vi "ADVM - AC Characteristics 2 Channel Measurements.vi"() -> ()   [LabVIEW 2021]
uses:
  <vilib>/PDM Acquisition Toolkit/shared/controls/i2s frame size.ctl
  <vilib>/PDM Acquisition Toolkit/shared/controls/PCM Data Format Configuration.ctl
  <vilib>/PDM Acquisition Toolkit/shared/controls/Digital Edge.ctl
  <vilib>/PDM Acquisition Toolkit/shared/controls/PCM Bit Endianness.ctl
  <vilib>/PDM Acquisition Toolkit/shared/controls/PCM Data Justification.ctl
  <vilib>/PDM Acquisition Toolkit/shared/controls/PCM Frame Sync Control.ctl
  <vilib>/PDM Acquisition Toolkit/host/Classes/Tasks/PDM Tasks/Controls/Acquisition Mode.ctl
  <vilib>/addons/_NISVFA/_Shared subVIs/Controls/svc_Window.ctl
  <vilib>/addons/_NISVFA/_Shared subVIs/Common/SVL Set dB Reference (N Ch - 1 Ref).vi
  <vilib>/addons/Sound and Vibration/svt_Level/SVL AC & DC Level (Time) (N Ch).vi
  <vilib>/addons/Sound and Vibration/svt_Single Tone Measurements/SVT Spurious Free Dynamic Range (Frequency) (1 Ch).vi
  <vilib>/addons/_NISVFA/_Spectrum Processing/SVFA Unit Conversion (Complex) (1 Ch).vi
  <vilib>/addons/_NISVFA/_Spectrum Processing/SVFA Get Spectrum Subset (1 Ch).vi
  <vilib>/addons/_NISVFA/_Shared subVIs/Common/SVL Set dB Reference (1 Ch).vi
  <vilib>/addons/Sound and Vibration/svt_Level/SVL AC & DC Level (Time) (1 Ch).vi
  <vilib>/addons/_NISVFA/_Spectrum Processing/SVFA Get Spectrum Subset (Complex) (1 Ch).vi
  <vilib>/addons/_NISVFA/_Shared subVIs/Common/svc_Window Parameters.vi
  <vilib>/addons/_NISVFA/_Shared subVIs/Common/svc_Extract Single Tone Information (complex).vi
  <vilib>/addons/_NISVFA/_Shared subVIs/Common/svc_Check Frequency Range in Spectrum.vi
  <vilib>/addons/_NISVFA/_Spectrum Processing/SVFA Spectrum Peak Search.vi
  <vilib>/addons/_NISVFA/_Spectrum Processing/SVFA Spectrum Peak Search (1 Ch).vi
  <vilib>/addons/_NISVFA/_Shared subVIs/Common/svc_Spectrum Units.vi
  <vilib>/addons/_NISVFA/_Shared subVIs/Common/svc_Log View for Spectrum (1Ch).vi
  <vilib>/addons/_NISVFA/_Spectrum Processing/SVFA Unit Conversion (1 Ch).vi
  <vilib>/addons/_NISVFA/_Shared subVIs/Common/svc_Complex Datatype Defaults.vi
  <vilib>/addons/_NISVFA/_Shared subVIs/Common/svc_Build Unit Label for Frequency Range.vi
  <vilib>/addons/_NISVFA/_Shared subVIs/Common/SVL Set dB Reference (variant).vi
  <vilib>/addons/_NISVFA/_Shared subVIs/Common/svc_Get SV Channel Info.vi
  <vilib>/Analysis/baseanly.llb/Mean.vi
  <vilib>/Analysis/baseanly.llb/Mean (DBL).vi
  <vilib>/addons/_NISVFA/_Shared subVIs/Windowing/svfa_Scaled Time Domain Window (Array).vi
  <vilib>/addons/_NISVFA/_Spectrum Processing/SVFA Get Tone Amplitude and Phase (1 Ch).vi
  <vilib>/addons/_NISVFA/_Spectrum Processing/subVIs/svfa_Compute Complex Spectrum for Export.vi
  <vilib>/addons/_NISVFA/_Shared subVIs/Common/svc_Check Frequency Range in Bandwidth.vi
  <vilib>/addons/_NISVFA/_Shared subVIs/Common/svc_Convert Start and Stop to Start Index and Length.vi
  <vilib>/addons/_NISVFA/_Spectrum Processing/subVIs/svfa_Spectrum Peak Search.vi
  <vilib>/addons/_NISVFA/_Shared subVIs/Common/svc_Format Value (DBL).vi
  <vilib>/addons/_NISVFA/_Shared subVIs/Common/svc_Get Weighting Enum and Labels.vi
  <vilib>/addons/_NISVFA/_Shared subVIs/Common/svc_Engineering Units to Unit Label.vi
  <vilib>/addons/_NISVFA/_Shared subVIs/Common/svc_Surround NonAlpha String with Parentheses.vi
  <vilib>/dlg_ctls.llb/Space Constant.vi
  <vilib>/addons/_NISVFA/_Shared subVIs/Common/svc_Unwrap Phase.vi
  <vilib>/addons/_NISVFA/_Shared subVIs/Common/svc_Convert Spectrum Array to dB.vi
  <vilib>/addons/_NISVFA/_Spectrum Processing/subVIs/svfa_Conversion Utility (spectrum info).vi
  <vilib>/addons/_NISVFA/_Shared subVIs/Common/svc_Unit Label to Engineering Units.vi
  <vilib>/addons/_NISVFA/_Spectrum Processing/subVIs/svfa_Spectrum Info Window to windowTd Type Def.vi
  <vilib>/Analysis/4window.llb/Force Window.vi
  <vilib>/Analysis/4window.llb/Force Window (DBL).vi
  <vilib>/Analysis/4window.llb/Exponential Window.vi
  <vilib>/Analysis/4window.llb/Exponential Window (DBL).vi
  <vilib>/addons/_NISVFA/_Spectrum Processing/subVIs/svfa_Window Frequency Response.vi
  <vilib>/addons/_NISVFA/_Spectrum Processing/subVIs/svfa_Window Frequency Response (double array).vi
  <vilib>/Analysis/baseanly.llb/Dot Product.vi
  <vilib>/Analysis/baseanly.llb/Complex Dot Product.vi
  <vilib>/addons/_NISVFA/_Spectrum Processing/subVIs/svfa_Peak Rough Search Indices.vi
  <vilib>/addons/_NISVFA/_Shared subVIs/Common/svc_Unit Label Lexical Class.vi
  <vilib>/addons/_NISVFA/_Spectrum Processing/subVIs/svfa_Peak to RMS to Peak2Peak.vi
  <vilib>/addons/_NISVFA/_Spectrum Processing/subVIs/svfa_Mag to Mag2.vi
  <vilib>/addons/_NISVFA/_Spectrum Processing/subVIs/svfa_Linear to dB.vi
  <vilib>/addons/_NISVFA/_Spectrum Processing/subVIs/svfa_dBrefA to dBrefB.vi
  <vilib>/addons/_NISVFA/_Spectrum Processing/subVIs/svfa_Spectrum to Spectral Density.vi
  <vilib>/addons/_NISVFA/_Spectrum Processing/subVIs/svfa_Rect Window Frequency Response.vi
  <vilib>/addons/_NISVFA/_Spectrum Processing/subVIs/svfa_Cosine Window Coefficients.vi
  <vilib>/PDM Acquisition Toolkit/host/API/Public/Create Tasks/Create PCM Input Task.vi
  <vilib>/PDM Acquisition Toolkit/host/API/Public/Configure/Timing/Configure Timing - PCM Input Slave.vi
  <vilib>/PDM Acquisition Toolkit/host/API/Public/Configure/PDM Channel/Configure Microphone Sensitivity FSPA - PCM Input Task.vi
  <vilib>/DAQmx/create/channels.llb/DAQmx Create Channel (AO-FuncGen).vi
  <vilib>/PDM Acquisition Toolkit/host/API/Public/Commit/Commit PCM Input Task.vi
  <vilib>/PDM Acquisition Toolkit/host/API/Public/Start/Start PCM Input Task.vi
  <vilib>/PDM Acquisition Toolkit/host/API/Public/Read/Read PCM Input Waveform.vi
  <vilib>/PDM Acquisition Toolkit/host/API/Public/Clear/Clear PCM Input Task.vi
  <vilib>/addons/Sound and Vibration/svt_Weighting/SVT Weighting Filter (N Ch).vi
  <vilib>/addons/_NISVFA/_Shared subVIs/Common/svc_Caller VI Returned in Error Source.vi
  <vilib>/addons/_NISVFA/_Shared subVIs/Common/svc_Get Window Info.vi
  <vilib>/Analysis/0measdsp.llb/Scaled Time Domain Window.vi
  <vilib>/Analysis/0measdsp.llb/Scaled Time Domain Window (DBL).vi
  <vilib>/Utility/error.llb/Error Cluster From Error Code.vi
  <vilib>/Analysis/baseanly.llb/Std Deviation and Variance.vi
  <vilib>/addons/Sound and Vibration/svt_Single Tone Measurements/SVT Gain (Time) (1 Ch).vi
  <vilib>/addons/Sound and Vibration/svt_Distortion/SVT SNR without Harmonics (Frequency) (1 Ch).vi
  <vilib>/addons/Sound and Vibration/svt_Single Tone Measurements/SVT Dynamic Range (Frequency) (1 Ch).vi
  <vilib>/addons/Sound and Vibration/svt_Distortion/subVIs/sv_Check Data Valid (Audio) (1 Ch).vi
  <vilib>/addons/_NISVFA/_Shared subVIs/Common/svc_Convert Frequency to Frequency String.vi
  <vilib>/Analysis/4window.llb/window parameters.vi
  <vilib>/Analysis/4window.llb/Window Properties.vi
  <vilib>/Analysis/4window.llb/Window Properties by Name.vi
  <vilib>/addons/_NISVFA/_Spectrum Processing/subVIs/svfa_Spectrum Peak Tone Search and Estimation (complex).vi
  <vilib>/measure/masignal.llb/Tones and Noise Waveform.vi
  <vilib>/addons/_NISVFA/_Shared subVIs/Common/svc_FFT with Window.vi
  <vilib>/Analysis/1siggen.llb/Square Wave.vi
  <vilib>/addons/_NISVFA/_Spectrum Processing/subVIs/svfa_Three Finger Peak Search.vi
  <vilib>/addons/Sound and Vibration/svt_Distortion/subVIs/sv_Peak View Amplitude (1 Ch).vi
  <vilib>/PDM Acquisition Toolkit/host/Classes/Tasks/PDM Tasks/PDM Task.lvclass
  <vilib>/PDM Acquisition Toolkit/host/API/PDM Acquisition Toolkit.lvlib
  <vilib>/addons/Sound and Vibration/svt_Single Tone Measurements/SoundVib_SingleTone.lvlib
  <vilib>/addons/Sound and Vibration/svt_Distortion/SoundVib_Distortion.lvlib
  <vilib>/PDM Acquisition Toolkit/shared/PDM Shared.lvlib
  <vilib>/addons/Sound and Vibration/svt_Weighting/SoundVib_ABCWeighting.lvlib
  <vilib>/PDM Acquisition Toolkit/host/API/Public/Configure/Timing/Configure Timing - I2S Input Slave.vi
  <vilib>/PDM Acquisition Toolkit/host/API/Public/Create Tasks/Create I2S Input Task.vi
  <vilib>/PDM Acquisition Toolkit/host/Classes/Tasks/I2S Input/I2S Input Task.lvclass
  <vilib>/PDM Acquisition Toolkit/host/Classes/Tasks/PCM Input/PCM Input Task.lvclass
panel:
  in  "DSG resource name":string="4468/ao0:1"
  in  "WEIGHTING":T1(ring)
  in  "DUT FULL SCALE":dbl=3.16 format="%.3p"
  out "error out":errorcluster
  out "Sampling Rate":dbl=192000.0 format="%#_6p"
  out "MeasTable":string[][](table)
  in  "I2S Number of Words":u32=19200 caption="NO OF WORDS"
  in  "I2S Word Length":u32=24 caption="WORD LENGTH"
  in  "I2S Clock Rate":u32=12288000 caption="CLOCK RATE"
  in  "THD Maximum Harmonic":u32=9 caption="MAX HARMONIC"
  in  "Measurement Band Stop":dbl=20000.0 caption="BAND STOP" format="%#_6pHz"
  in  "Measurement Band Start":dbl=20.0 caption="BAND START" format="%#_6pHz"
  in  "DSG amplitude":dbl=1.0 caption="AMPLITUDE" format="%#_6pV"
  in  "DSG frequency":dbl=1000.0 caption="FREQUENCY" format="%#_6pHz"
  in  "Mic sensitivity (FS/Pa)":dbl=0.34762 caption="SENSITIVITY" format="%.3fFS/Pa"
  in  "I2S Channel List":string="7820\\PCMi 0" caption="CHANNEL LIST"
  out "MeasGraphs":enum32{"Frequency Domain", "Time Domain"}(tab)
  out "FrequencyDomain":cluster{"x0":dbl, "dx":dbl, "magnitude":dbl[]}[](graph) caption="AC"
  out "TimeDomain":waveform(dbl)[](graph) caption="AC"
  # "Measurement"
  # "Analog Source"
  # "Protocol Setting"
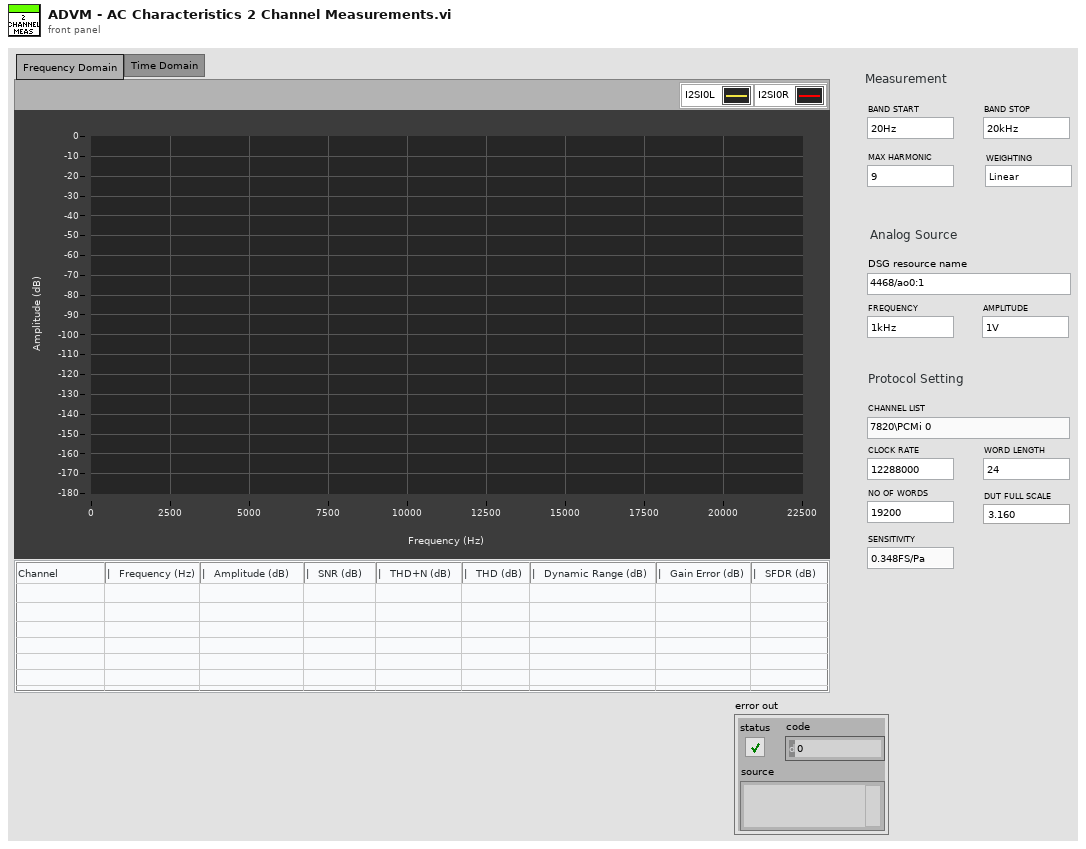
[diagram p1: front panel]
types:
  T1 = enum16{"Linear", "A-weighting", "B-weighting", "C-weighting"}
  T2 = cluster{"band start (Hz)":dbl, "band stop (Hz)":dbl}
  T3 = typedef "PDM Shared.lvlib/i2s frame size.ctl" = enum16{"32bits", "64bits"}
  T4 = cluster{"frequency range":cluster{"band start (Hz)":dbl, "band stop (Hz)":dbl}, "THD maximum harmonic":i32, "amplitude":dbl, "frequency (Hz)":dbl, "microphone sensitivity (FS/Pa)":dbl, "number of words":i32, "channel list":string, "logic level":enum16{"3.3 V", "1.8 V", "1.2 V"}, "I2S serial clock rate 2":u32, "frame size":T3, "word length":u32, "Data Latch at SCK cycle":u8, "Playback .WAV File?":bool, "Record .WAV File?":bool, "Record wave file path":path, "Playback .WAV file path":path, "number of channels":i32, "DUT full scale (V pk)":dbl, "output channel":tag[]}
  T5 = typedef "PDM Shared.lvlib/PCM Frame Sync Control.ctl" = cluster{"Frame Length":u16, "Frame Sync Pulse Width":u16, "Bit Clock Edge  Sync":T6}
  T6 = typedef "PDM Shared.lvlib/Digital Edge.ctl" = enum8{"Rising", "Falling"}
  T7 = typedef "PDM Shared.lvlib/PCM Data Format Configuration.ctl" = cluster{"Frame Sync Edge for Channel 0":T6, "Channel Count Per Frame":u8, "Channel Length":u16, "Bit Depth":u8, "Channel 0 Offset":u16, "Endianness":T8, "Data Justification":T9}
  T8 = typedef "PDM Shared.lvlib/PCM Bit Endianness.ctl" = enum16{"MSB First", "LSB First"}
  T9 = typedef "PDM Shared.lvlib/PCM Data Justification.ctl" = enum16{"Left Justified", "Right Justified"}
  T10 = typedef "PDM Acquisition Class Library.lvlib/PDM Task.lvclass/Acquisition Mode.ctl" = enum16{"Finite", "Continuous"}
  T11 = cluster{"linear/dB":enum16{"no change", "linear", "dB"}, "dB reference (0: no change)":dbl, "power/magnitude":enum16{"no change", "power", "magnitude"}, "view":enum16{"no change", "rms", "peak", "peak-peak"}}
  T12 = enum16{"no change", "spectrum", "spectral density"}
  T13 = cluster{"gain units":enum16{"dB", "linear ratio"}, "detected fundamental amplitude units":enum16{"EU rms", "EU peak", "EU peak-peak"}}
  T14 = cluster{"SNR units":enum16{"dB", "linear ratio", "%"}, "detected fundamental amplitude units":enum16{"EU rms", "EU peak", "EU peak-peak"}}
  T15 = typedef "PDM Acquisition Class Library.lvlib/I2S Input Task.lvclass/DVR I2S Input Task.ctl" = refnum<data-value>
  T16 = typedef "PDM Acquisition Class Library.lvlib/PCM Input Task.lvclass/DVR PCM Input Task.ctl" = refnum<data-value>
  T17 = typedef "svc_Window.ctl" = u32
  T18 = typedef "svc_Spectrum Info.ctl" = cluster{"channel name":string, "description":string, "x-axis units":T19, "spectral info":cluster{"spectrum type":T20, "linear/dB":enum16{"linear", "dB"}, "window":u16, "window size":i32, "FFT size":i32}, "engineering units":T21, "custom label":string, "dB reference [EU]":dbl, "peak units":enum16{"rms", "peak", "peak-peak"}, "weighting filter":T22, "spectral density?":bool, "unit label":string, "spectrum skewed?":bool, "complimentary spectrum units":T23}
  T19 = typedef "svc_X-Axis Units.ctl" = u16
  T20 = typedef "svc_Spectrum Type.ctl" = enum16{"FFT Spectrum [complex]", "Amplitude [Magnitude]", "Power [Magnitude^2]", "Cross Spectrum [complex]", "Frequency Response [Complex]"}
  T21 = typedef "svc_Engineering Units Text Ring.ctl" = u16
  T22 = typedef "svc_Weighting Filter Text Ring.ctl" = u16
  T23 = typedef "svc_Complimentary Spectrum Units.ctl" = enum16{"none", "radians", "degrees", "cycles", "imaginary"}
  T24 = cluster{"complex spectrum response":cluster{"f0":dbl, "df":dbl, "complex spectrum":cdb[]}, "spectrum info":T18}
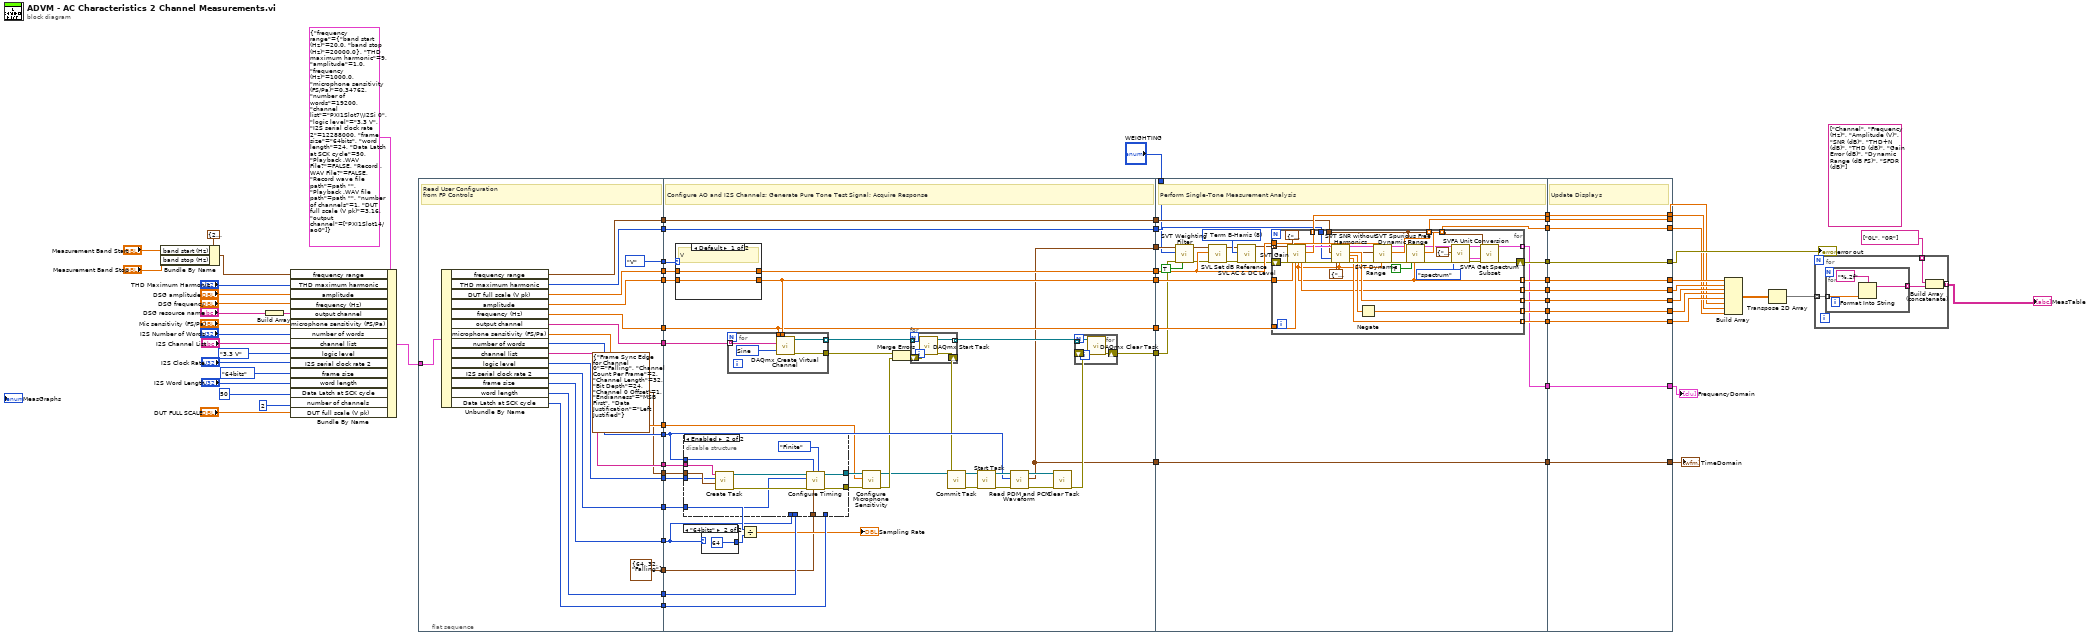
[diagram p0: block diagram]
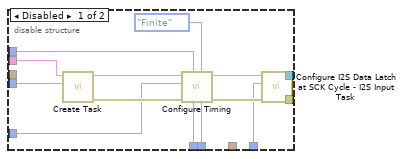
[diagram p2: hidden frame]
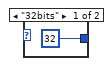
[diagram p3: hidden frame]
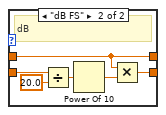
[diagram p4: hidden frame]
diagram:
  (unwired) string[] ["Channel", "Frequency (Hz)", "Amplitude (V)", "SNR (dB)", "THD+N (dB)", "THD (dB)", "Gain Error (dB)", "Dynamic Range (dB FS)", "SFDR (dB)"] ("MeasTable")
  n1 = Bundle By Name(cluster=T2 {"band start (Hz)"=20.0, "band stop (Hz)"=20000.0} ("frequency range"), "band start (Hz)"="Measurement Band Start", "band stop (Hz)"="Measurement Band Stop") -> (w39:T2)
  n2 = Build Array("DSG resource name") -> (w6:string[])
  n3 = Bundle By Name(cluster=T4 {"frequency range"={"band start (Hz)"=20.0, "band stop (Hz)"=20000.0}, "THD maximum harmonic"=9, "amplitude"=1.0, "frequency (Hz)"=1000.0, "microphone sensitivity (FS/Pa)"=0.34762, "number of words"=19200, "channel list"="PXI1Slot7\\I2Si 0", "logic level"=enum."3.3 V", "I2S serial clock rate 2"=12288000, "frame size"=enum."64bits", "word length"=24, "Data Latch at SCK cycle"=50, "Playback .WAV File?"=FALSE, "Record .WAV File?"=FALSE, "Record wave file path"=path "", "Playback .WAV file path"=path "", "number of channels"=1, "DUT full scale (V pk)"=3.16, "output channel"=["PXI1Slot14/ao0"]}, "frequency range"=w39, "THD maximum harmonic"="THD Maximum Harmonic", "amplitude"="DSG amplitude", "frequency (Hz)"="DSG frequency", "output channel"=w6, "microphone sensitivity (FS/Pa)"="Mic sensitivity (FS/Pa)", "number of words"="I2S Number of Words", "channel list"="I2S Channel List", "logic level"=enum16{"3.3 V", "1.8 V", "1.2 V"}."3.3 V" ("I2S Logic Level"), "I2S serial clock rate 2"="I2S Clock Rate", "frame size"=enum16{"32bits", "64bits"}."64bits" ("I2S Frame Size"), "word length"="I2S Word Length", "Data Latch at SCK cycle"=u8 50 ("I2S Data Latch at SCK Cycle"), "number of channels"=2, "DUT full scale (V pk)"="DUT FULL SCALE") -> (w26:T4)
  n4 = flat-sequence {
    tunnel: [w88] -> w73
    tunnel: [w85] -> w72
    tunnel: [w84] -> w71
    tunnel: [w87] -> w70
    tunnel: [w86] -> w69
    tunnel: [enum16{"V", "dB FS"}."V" ("amplitude units")] -> w68
    tunnel: [w79] -> w67
    tunnel: [w80] -> w66
    tunnel: [w76] -> w65
    tunnel: [w82] -> w64
    tunnel: [w77] -> w63
    tunnel: [w78] -> w62
    tunnel: [w81] -> w61
    tunnel: [w83] -> w45
    tunnel: w26 -> [w90]
    tunnel: [w89] -> w25
    tunnel: [T7 {"Frame Sync Edge for Channel 0"=enum."Falling", "Channel Count Per Frame"=2, "Channel Length"=32, "Bit Depth"=24, "Channel 0 Offset"=1, "Endianness"=enum."MSB First", "Data Justification"=enum."Left Justified"} ("PCM data configuration")] -> w2
    tunnel: [T5 {"Frame Length"=64, "Frame Sync Pulse Width"=32, "Bit Clock Edge  Sync"=enum."Falling"} ("Frame Sync Clock Control")] -> w1
    tunnel: w73 -> [w126]
    tunnel: w72 -> [w119]
    tunnel: w71 -> [w124]
    tunnel: w70 -> [w129]
    tunnel: w69 -> [w128]
    tunnel: w68 -> [w125]
    tunnel: [w130] -> w60
    tunnel: [w127] -> w59
    tunnel: [w126] -> w58
    tunnel: [w123] -> w57
    tunnel: [w119] -> w56
    tunnel: [w99] -> w55
    tunnel: [w117] -> w54
    tunnel: w67 -> [w109]
    tunnel: w66 -> [w108]
    tunnel: w65 -> [w107]
    tunnel: w64 -> [w106]
    tunnel: w63 -> [w105]
    tunnel: w62 -> [w104]
    tunnel: w61 -> [w103]
    tunnel: w45 -> [w96]
    tunnel: w25 -> [w130]
    tunnel: [w99] -> w21
    tunnel: w2 -> [w93]
    tunnel: w1 -> [w92]
    tunnel: [w200] -> w53
    tunnel: [w199] -> w52
    tunnel: [w190] -> w51
    tunnel: [w198] -> w50
    tunnel: [w197] -> w49
    tunnel: [w196] -> w48
    tunnel: [w195] -> w47
    tunnel: [w189] -> w46
    tunnel: w60 -> [w188]
    tunnel: w59 -> [w202]
    tunnel: w58 -> [w193]
    tunnel: w57 -> [w201]
    tunnel: w56 -> [w194]
    tunnel: w55 -> [w186]
    tunnel: w54 -> [w184]
    tunnel: [w191] -> w22
    tunnel: w21 -> [w191]
    tunnel: [w187] -> w20
    tunnel: "WEIGHTING" -> [w182]
    tunnel: [w179] -> w4
    tunnel: w53 -> [w243]
    tunnel: w52 -> [w242]
    tunnel: w51 -> [w250]
    tunnel: w50 -> [w244]
    tunnel: w49 -> [w245]
    tunnel: w48 -> [w246]
    tunnel: w47 -> [w247]
    tunnel: w46 -> [w248]
    tunnel: [w250] -> w44
    tunnel: [w249] -> w23
    tunnel: w22 -> [w249]
    tunnel: w20 -> [w241]
    tunnel: [w248] -> w19
    tunnel: [w247] -> w18
    tunnel: [w246] -> w17
    tunnel: [w245] -> w16
    tunnel: [w244] -> w15
    tunnel: [w243] -> w14
    tunnel: [w242] -> w13
    tunnel: [w241] -> w12
    tunnel: w4 -> [w240]
    tunnel: [w240] -> w3
    frame #0 {
      # "Read User Configuration\nfrom FP Controls"
      n5 = Unbundle By Name(w90) -> ("frequency range"=w89:T2, "THD maximum harmonic"=w88:i32, "DUT full scale (V pk)"=w87:dbl, "amplitude"=w86:dbl, "frequency (Hz)"=w85:dbl, "output channel"=w84:tag[], "microphone sensitivity (FS/Pa)"=w83:dbl, "number of words"=w82:i32, "channel list"=w81:string, "logic level"=w80:enum16{"3.3 V", "1.8 V", "1.2 V"}, "I2S serial clock rate 2"=w79:u32, "frame size"=w78:T3, "word length"=w77:u32, "Data Latch at SCK cycle"=w76:u8)
    }
    frame #1 {
      # "Configure AO and I2S Channels; Generate Pure Tone Test Signal; Acquire Response"
      n6 = case shown="Default" w125 {
        tunnel: [w172 w174] -> w123
        tunnel: w128 -> [w172 w178]
        tunnel: w129 -> [w171 w173]
        tunnel: [w171 w173] -> w127
        frame Default {
          # "V"
        }
        frame "dB FS" {
          # "dB"
          n7 = Divide(x=w178, y=20.0) -> (x/y=w176:dbl)
          n8 = Power Of 10(x=w176) -> (10^x=w175:dbl)
          n9 = Multiply(x=w173, y=w175) -> (x*y=w174:dbl)
        }
      }
      n10 = disable-structure shown="Enabled" {
        disable-tunnel: [w140 w150] -> w98
        disable-tunnel: [w139 w151] -> w97
        disable-tunnel: w109 -> [w137 w148]
        disable-tunnel: w108 -> [w136 w146]
        disable-tunnel: w107 -> [w135 _]
        disable-tunnel: w106 -> [w134 w147]
        disable-tunnel: w105 -> [w133 _]
        disable-tunnel: w104 -> [w132 _]
        disable-tunnel: w103 -> [w131 w152]
        disable-tunnel: w93 -> [_ w149]
        disable-tunnel: w92 -> [_ w145]
        frame Disabled {
          n11 = call-poly <vilib>:"Create Task.vi"("logic level"=w136, "channel list"=w131) -> ("error out"=w143:errorcluster, "I2S input task out"=w142:T15)  [unwired: 8 in]
          n12 = call-poly <vilib>:"Configure Timing.vi"("word length"=w133, "acquisition mode"=Acquisition_Mode."Finite", "frame size"=w132, "number of words"=w134, "error in"=w143, "I2S serial clock rate"=w137, "I2S input task in"=w142) -> ("error out"=w141:errorcluster, "I2S input task out"=w138:T15)  [unwired: 3 in]
          n13 = call <vilib>:"Configure I2S Data Latch at SCK Cycle - I2S Input Task.vi"("error in"=w141, "data latch at SCK cycle"=w135, "I2S input task in"=w138) -> ("error out"=w140:errorcluster, "I2S input task out"=w139:T15)  [unwired: 7 in]
        }
        frame Enabled {
          n14 = call-poly <vilib>:"Create Task.vi"("PCM data configuration"=w149, "logic level"=w146, "channel list"=w152) -> ("error out"=w154:errorcluster, "PCM input task out"=w155:T16)  [unwired: 7 in]
          n15 = call-poly <vilib>:"Configure Timing.vi"("acquisition mode"=Acquisition_Mode."Finite", "Frame Sync Clock Control"=w145, "number of words per channel"=w147, "error in"=w154, "Bit Clock rate"=w148, "PCM input task in"=w155) -> ("error out"=w150:errorcluster, "PCM input task out"=w151:T16)  [unwired: 4 in]
        }
      }
      n16 = case shown="\"64bits\"" w104 {
        tunnel: [u8 32 ("frame size") u8 64 ("frame size")] -> w112
        frame "32bits" {
        }
        frame "64bits" {
        }
      }
      n17 = for {
        tunnel: w124 -> [w168] mode=indexing
        tunnel: w123 -> [w167]
        tunnel: [w166] -> w122
        tunnel: [w165] -> w120 mode=indexing
        tunnel: w119 -> [w164]
        w163 = 14751 items=["Sine"=14751, "Triangle"=14752, "Square"=14753, "Sawtooth"=14754] ("type")
        n18 = call-poly <vilib>:"DAQmx Create Virtual Channel.vi"("frequency"=w164, "amplitude"=w167, "physical channels"=w168, "type"=w163) -> ("task out"=w165:refnum<k21>, "error out"=w166:errorcluster)  [unwired: 10 in]
      }
      n19 = Divide(x=w109, y=w112) -> (x/y=→"Sampling Rate":dbl)
      n20 = call-poly <vilib>:"Configure Microphone Sensitivity.vi"("error in"=w98, "microphone sensitivity (FS/Pa)"=w96, "PCM input task in"=w97) -> ("error out"=w95:errorcluster, "PCM input task out"=w94:T16)  [unwired: 7 in]
      n21 = Merge Errors(w122, w95) -> (w121:errorcluster)
      n22 = for {
        tunnel: w120 -> [w161] mode=indexing
        tunnel: [w160] -> w118 mode=indexing
        shift-right: [w159] -> w102
        shift-left: w121 -> [w162]
        n23 = call <vilib>:"DAQmx Start Task.vi"("task/channels in"=w161, "error in"=w162) -> ("task out"=w160:refnum<k21>, "error out"=w159:errorcluster)  [unwired: 12 in]
      }
      n24 = call-poly <vilib>:"Commit Task.vi"("error in"=w102, "PCM input task in"=w94) -> ("error out"=w111:errorcluster, "PCM input task out"=w110:T16)  [unwired: 8 in]
      n25 = call-poly <vilib>:"Start Task.vi"("error in"=w111, "PCM input task in"=w110) -> ("error out"=w116:errorcluster, "PCM input task out"=w115:T16)  [unwired: 8 in]
      n26 = call-poly <vilib>:"Read PDM and PCM Waveform.vi"("error in"=w116, "words per channel"=w106, "PCM input task In"=w115) -> ("error out"=w114:errorcluster, "PCM waveforms"=w99:waveform(dbl)[], "PCM input task out"=w113:T16)  [unwired: 5 in, 1 out]
      n27 = call-poly <vilib>:"Clear Task.vi"("error in"=w114, "PCM input task in"=w113) -> ("error out"=w101:errorcluster)  [unwired: 9 in]
      n28 = for {
        tunnel: w118 -> [w158] mode=indexing
        shift-right: [w157] -> w117
        shift-left: w101 -> [w156]
        n29 = call <vilib>:"DAQmx Clear Task.vi"("task in"=w158, "error in"=w156) -> ("error out"=w157:errorcluster)  [unwired: 13 in]
      }
    }
    frame #2 {
      w205 = T17 8 items=["None"=0, "Hanning"=1, "Hamming"=2, "Blackman-Harris"=3, "Exact Blackman"=4, "Blackman"=5, "Flat Top"=6, "4 Term B-Harris "=7, "7 Term B-Harris"=8, "Low Sidelobe"=9, "Force"=64, "Exponential"=65, "Blackman Nuttall"=11, "Triangle"=30, "Bartlett-Hanning"=31, "Bohman"=32, "Parzen"=33, "Welch"=34, "Kaiser"=60, "Dolph-Chebyshev"=61, "Gaussian"=62] ("window")
      # "Perform Single-Tone Measurement Analysis"
      n30 = call-poly <vilib>:"SVT Weighting Filter.vi"("reset filter (F)"=TRUE, "error in (no error)"=w184, "weighting"=w182, "scaled signals [EU]"=w186) -> ("error out"=w183:errorcluster, "weighted signals [EU]"=w185:waveform(dbl)[])  [unwired: 5 in]
      n31 = call-poly <vilib>:"SVL Set dB Reference.vi"("error in (no error)"=w183, "dB reference [EU]"=w202, "scaled signals in [EU]"=w185) -> ("error out"=w204:errorcluster, "scaled signals out [EU]"=w203:waveform(dbl)[])  [unwired: 7 in]
      n32 = call-poly <vilib>:"SVL AC & DC Level.vi"("scaled signals in [EU]"=w203, "window"=w205, "error in (no error)"=w204) -> ("AC signals [EU]"=w180:waveform(dbl)[], "error out"=w192:errorcluster)  [unwired: 11 in, 4 out]
      n33 = for {
        tunnel: w201 -> [w232]
        tunnel: [w231] -> w200 mode=indexing
        tunnel: [w229] -> w198 mode=indexing
        tunnel: [w228] -> w197 mode=indexing
        tunnel: [w227] -> w196 mode=indexing
        tunnel: [w226] -> w195 mode=indexing
        tunnel: w194 -> [w225]
        tunnel: w193 -> [w223]
        tunnel: [w219] -> w189 mode=indexing
        tunnel: w188 -> [w208]
        tunnel: [w217] -> w187 mode=indexing
        tunnel: w180 -> [w216] mode=indexing
        tunnel: w202 -> [w233]
        tunnel: [w230] -> w199 mode=indexing
        shift-right: [w209] -> w190
        shift-left: w192 -> [w222]
        tunnel: [w206] -> w179 mode=indexing
        n34 = call-poly <vilib>:"SVT Gain.vi"("scaled signal [EU]"=w216, "error in (no error)"=w222, "desired units"=T13 {"gain units"=enum."dB", "detected fundamental amplitude units"=enum."EU peak"}, "amplitude [EU peak]"=w232, "expected fundamental frequency [Hz]"=w225) -> ("detected fundamental\nfrequency [Hz]"=w219:dbl, "detected fundamental\namplitude"=w226:dbl, "complex spectrum"=w224:T24, "gain"=w231:dbl, "error out"=w239:errorcluster)  [unwired: 9 in, 1 out]
        n35 = call-poly <vilib>:"SVT SNR without Harmonics.vi"("complex spectrum"=w224, "frequency range"=w208, "maximum harmonic"=w223, "error in (no error)"=w239, "desired units"=T14 {"SNR units"=enum."dB", "detected fundamental amplitude units"=enum."EU rms"}, "expected fundamental frequency [Hz]"=w219) -> ("complex spectrum"=w237:T24, "SNR (without harmonics)"=w227:dbl, "SINAD"=w236:dbl, "THD"=w229:dbl, "error out"=w238:errorcluster)  [unwired: 6 in, 3 out]
        n36 = Negate(x=w236) -> (-x=w228:dbl)
        n37 = call-poly <vilib>:"SVT Dynamic Range.vi"("complex spectrum"=w237, "frequency range"=w208, "error in (no error)"=w238, "full scale amplitude [EU peak]"=w233, "expected fundamental\nfrequency [Hz]"=w219) -> ("dup complex spectrum"=w221:T24, "dynamic range"=w230:dbl, "error out"=w220:errorcluster)  [unwired: 9 in, 3 out]
        n38 = call-poly <vilib>:"SVT Spurious Free Dynamic Range.vi"("complex spectrum"=w221, "frequency range"=w208, "error in (no error)"=w220, "exclude harmonics"=TRUE, "expected fundamental\nfrequency [Hz]"=w219) -> ("complex spectrum"=w214:T24, "spurious free dynamic range"=w217:dbl, "error out"=w215:errorcluster)  [unwired: 7 in, 5 out]
        n39 = call-poly <vilib>:"SVFA Unit Conversion.vi"("complex spectrum"=w214, "desired scaling"=T11 {"linear/dB"=enum."dB", "dB reference (0: no change)"=0.0, "power/magnitude"=enum."magnitude", "view"=enum."peak-peak"}, "spectral density desired"=T12."spectrum", "error in (no error)"=w215) -> ("converted spectrum"=w212:cluster{"x0":dbl, "dx":dbl, "magnitude":dbl[]}, "spectrum info out"=w211:T18, "error out"=w210:errorcluster)  [unwired: 10 in, 3 out]
        n40 = call-poly <vilib>:"SVFA Get Spectrum Subset.vi"("spectrum"=w212, "range"=w208, "spectrum info"=w211, "error in (no error)"=w210) -> ("spectrum subset"=w206:cluster{"x0":dbl, "dx":dbl, "magnitude":dbl[]}, "error out"=w209:errorcluster)  [unwired: 10 in, 4 out]
      }
    }
    frame #3 {
      # "Update Displays"
    }
  }
  n41 = Build Array(w19, w18, w17, w16, w15, w14, w13, w12) -> (w11:dbl[][])
  n42 = Transpose 2D Array(2D array=w11) -> (transposed array=w9:dbl[][])
  n43 = for {
    tunnel: w9 -> [w254] mode=indexing
    tunnel: [w252] -> w8 mode=indexing
    tunnel: string[] ["0L", "0R"] ("format string") -> [w251] mode=indexing
    n44 = for {
      tunnel: w254 -> [w257] mode=indexing
      tunnel: [w255] -> w253 mode=indexing
      n45 = Format Into String(format string="%.2f", w257) -> (resulting string=w255:string)  [unwired: 2 in, 1 out]
    }
    n46 = Build Array (concatenate)(w251, w253) -> (w252:string[])
  }
  "MeasTable" <- w8
  "error out" <- w44
  "TimeDomain" <- w23
  "FrequencyDomain" <- w3
